vi "Vector Facade.vi"(0 "Data In":T4, 2 "Display State In":T2, 3 "Container State":T3) -> (6 "Data Out":T4, 7 "Display State Out":T2, 8 "Action":T1)   [LabVIEW 2018, in "Vector Function Generator.xctl"]
uses:
  Vector Function Generator.xctl
  Vector Data.ctl
  <vilib>/_xctls/Container State.ctl
  Vector State.ctl
  <vilib>/_xctls/Action.ctl
  <userlib>/_LAVAcr/User_Interface/XControls/Waveform_XControl/Waveform Control.xctl
  <userlib>/_OpenG.lib/comparison/comparison.llb/I32 Changed__ogtk.vi
  <userlib>/_OpenG.lib/comparison/comparison.llb/Boolean Changed__ogtk.vi
  <vilib>/_xctls/XControlSupport.lvlib
panel:
  in  "Order":u16(ring) items=["R then Theta", "Theta then R", "R and Theta"]
  in  "Tab Control":enum32{"R", "Theta", "Plot"}(tab)
  in  "R":waveform(dbl)(xcontrol)
  in  "Theta":waveform(dbl)(xcontrol)
  out "Polar Plot":picture
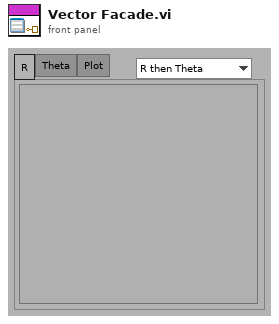
[diagram p1: front panel]
types:
  T1 = typedef "XControlSupport.lvlib/Action.ctl" = cluster{"Data Changed?":bool, "State Changed?":bool, "Action Name":string}
  T2 = typedef "Vector Function Generator.xctl/Vector State.ctl" = cluster{"Current Position":i32, "Show Current Position":bool, "Mode (F=Polar)":bool, "digits":i32, "sf(F) or dp ?":bool, "Units":string}
  T3 = typedef "XControlSupport.lvlib/Container State.ctl" = cluster{"Indicator?":bool, "Run Mode?":bool, " Refnum":refnum<vi>}
  T4 = typedef "Vector Function Generator.xctl/Vector Data.ctl" = waveform(cdb)
  T5 = typedef "Waveform Control.xctl/FP Controls.ctl" = cluster{"Type":T6, "Periods":dbl, "Points":i32, "Offset":dbl, "Amplitdue":dbl, "Phase":dbl, "func":string}
  T6 = typedef "Waveform Control.xctl/Function Types.ctl" = enum16{"Level", "Sine", "Triangle", "Ramp", "Saw Tooth", "Square", "Function"}
  T7 = typedef "LVRectTypeDef.ctl" = cluster{"Left":i16, "Top":i16, "Right":i16, "Bottom":i16}
  T8 = typedef "LVBoundsTypeDef.ctl" = cluster{"Width":u32, "Height":u32}
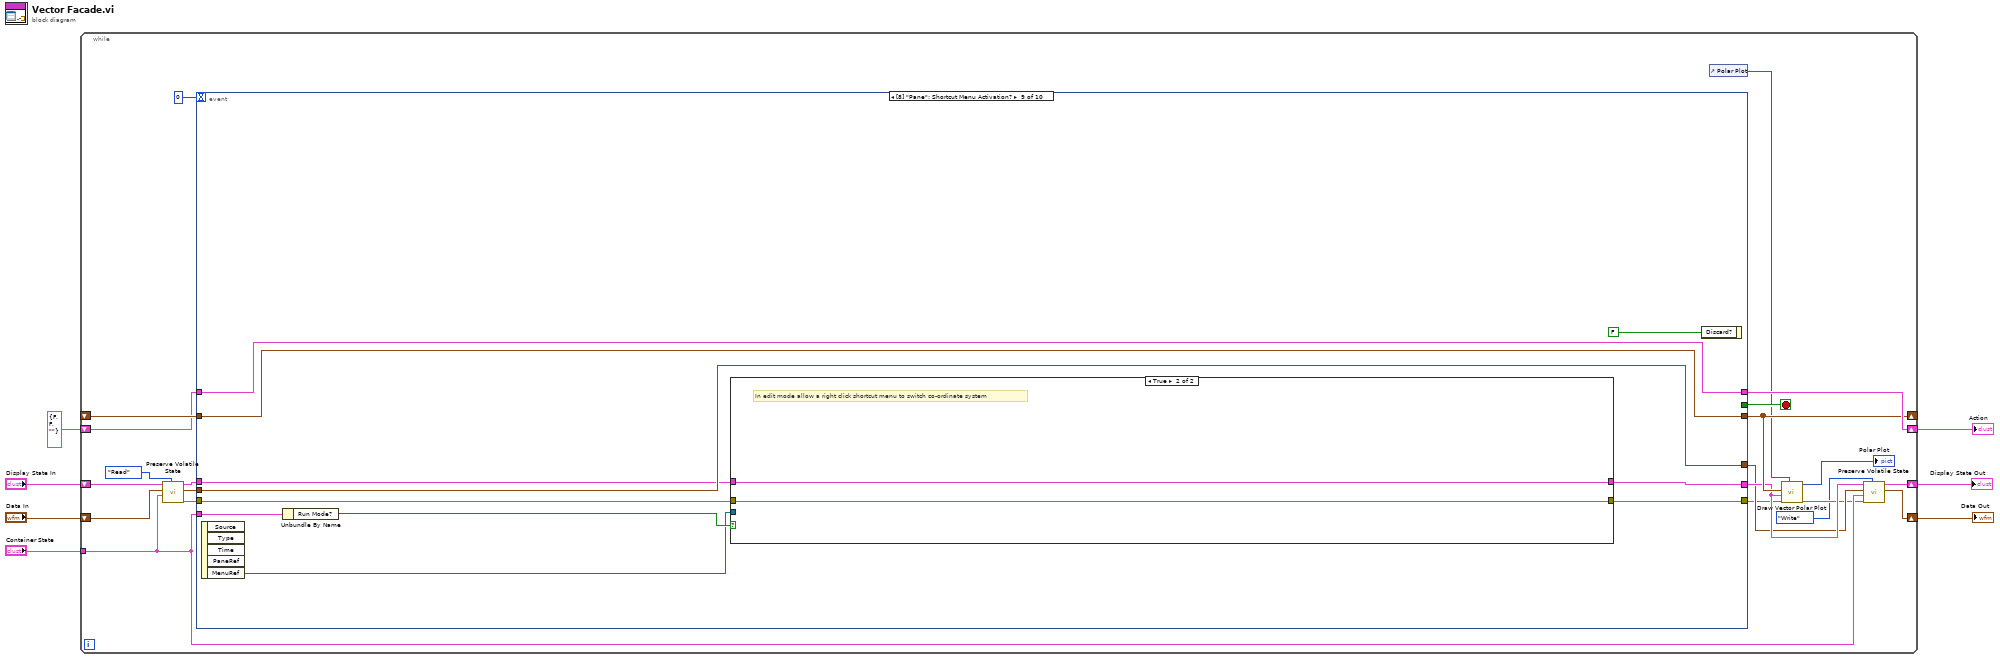
[diagram p0: block diagram]
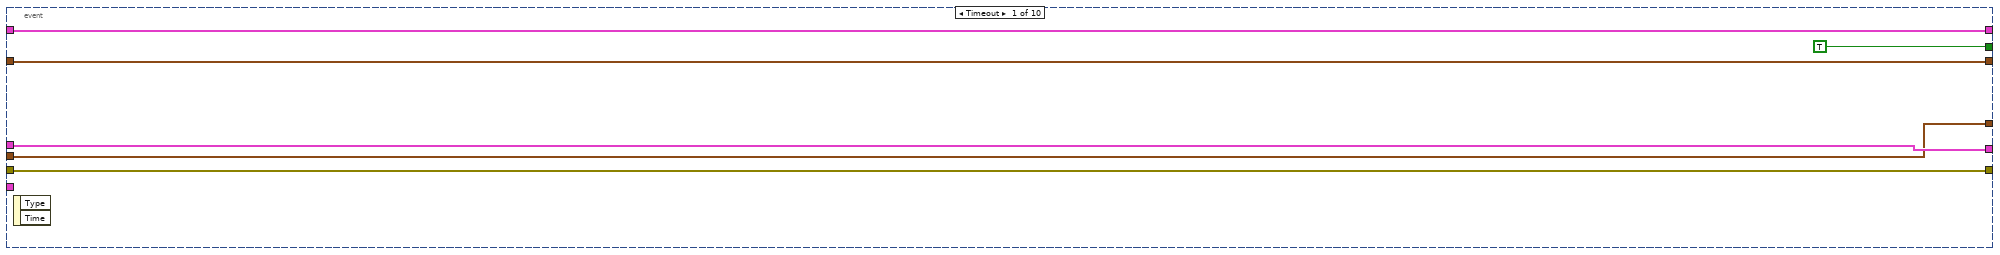
[diagram p2: hidden frame]
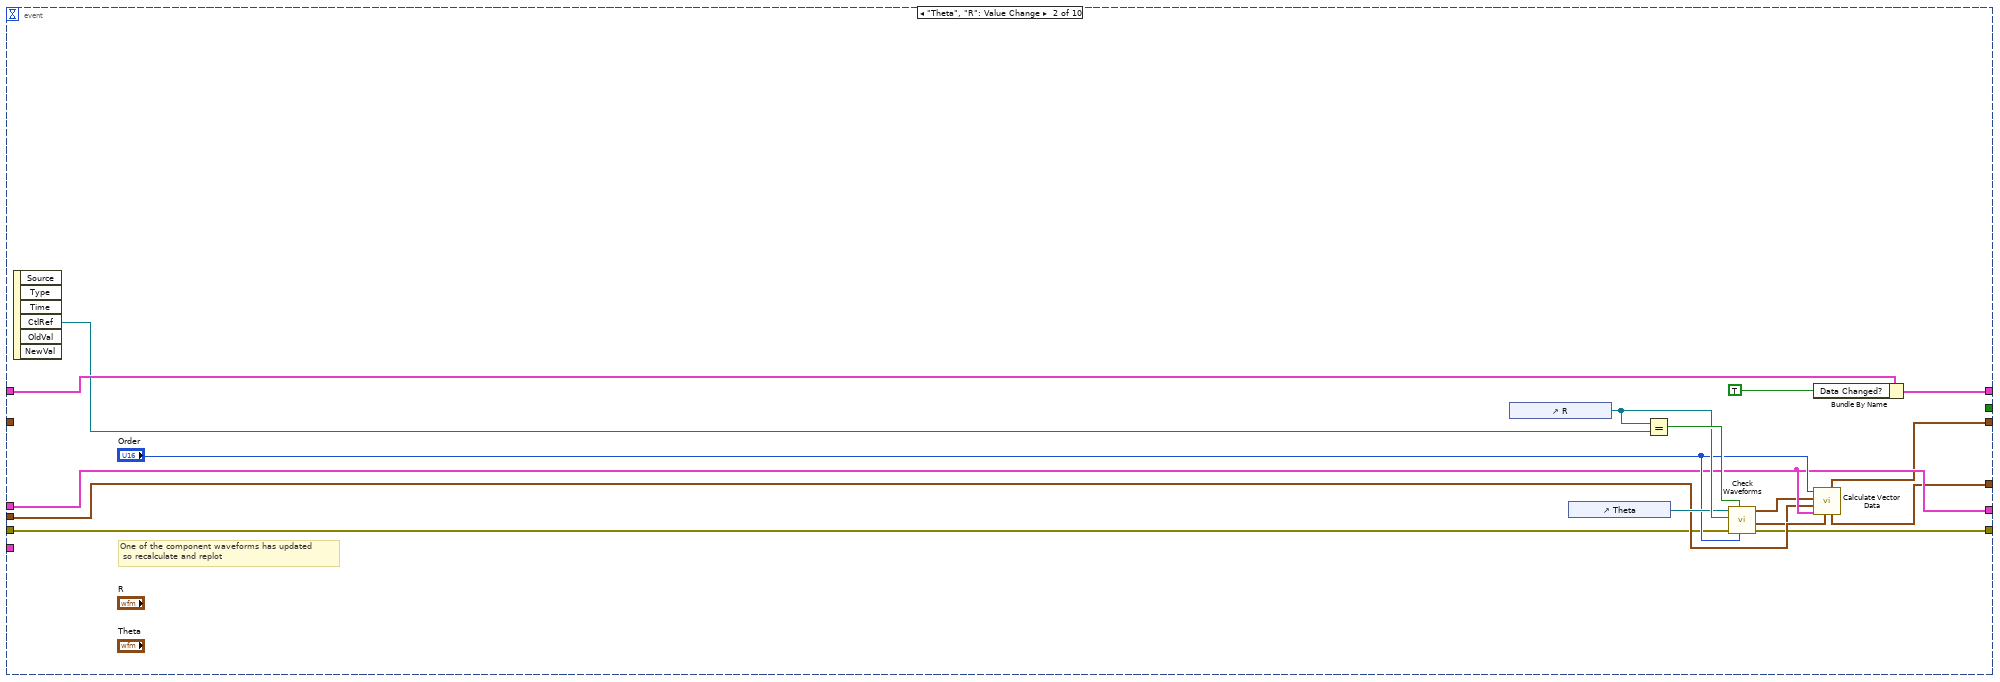
[diagram p3: hidden frame]
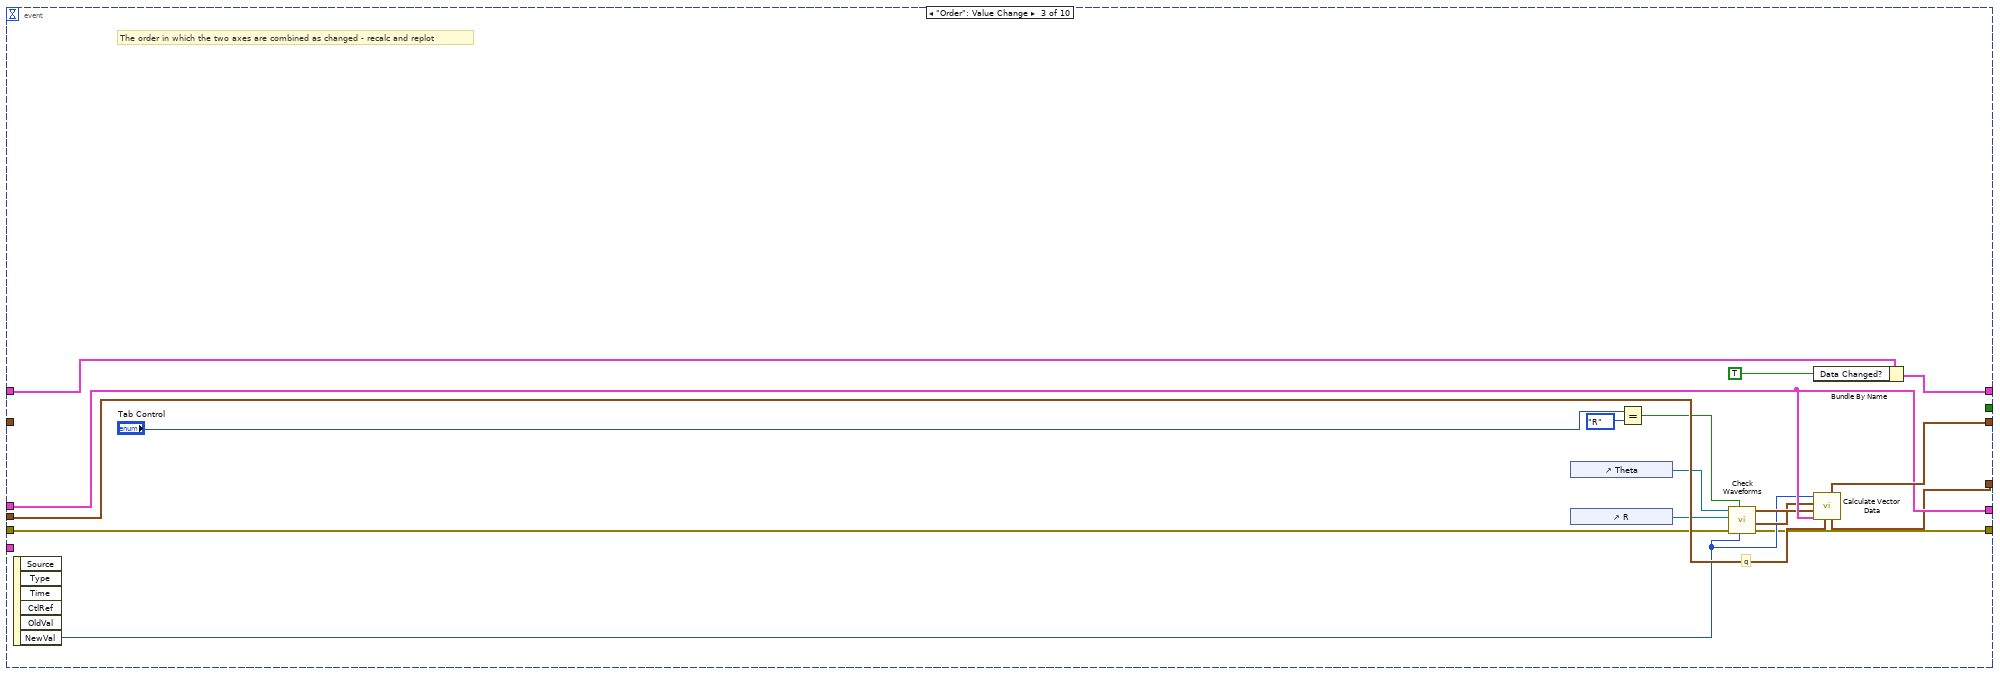
[diagram p4: hidden frame]
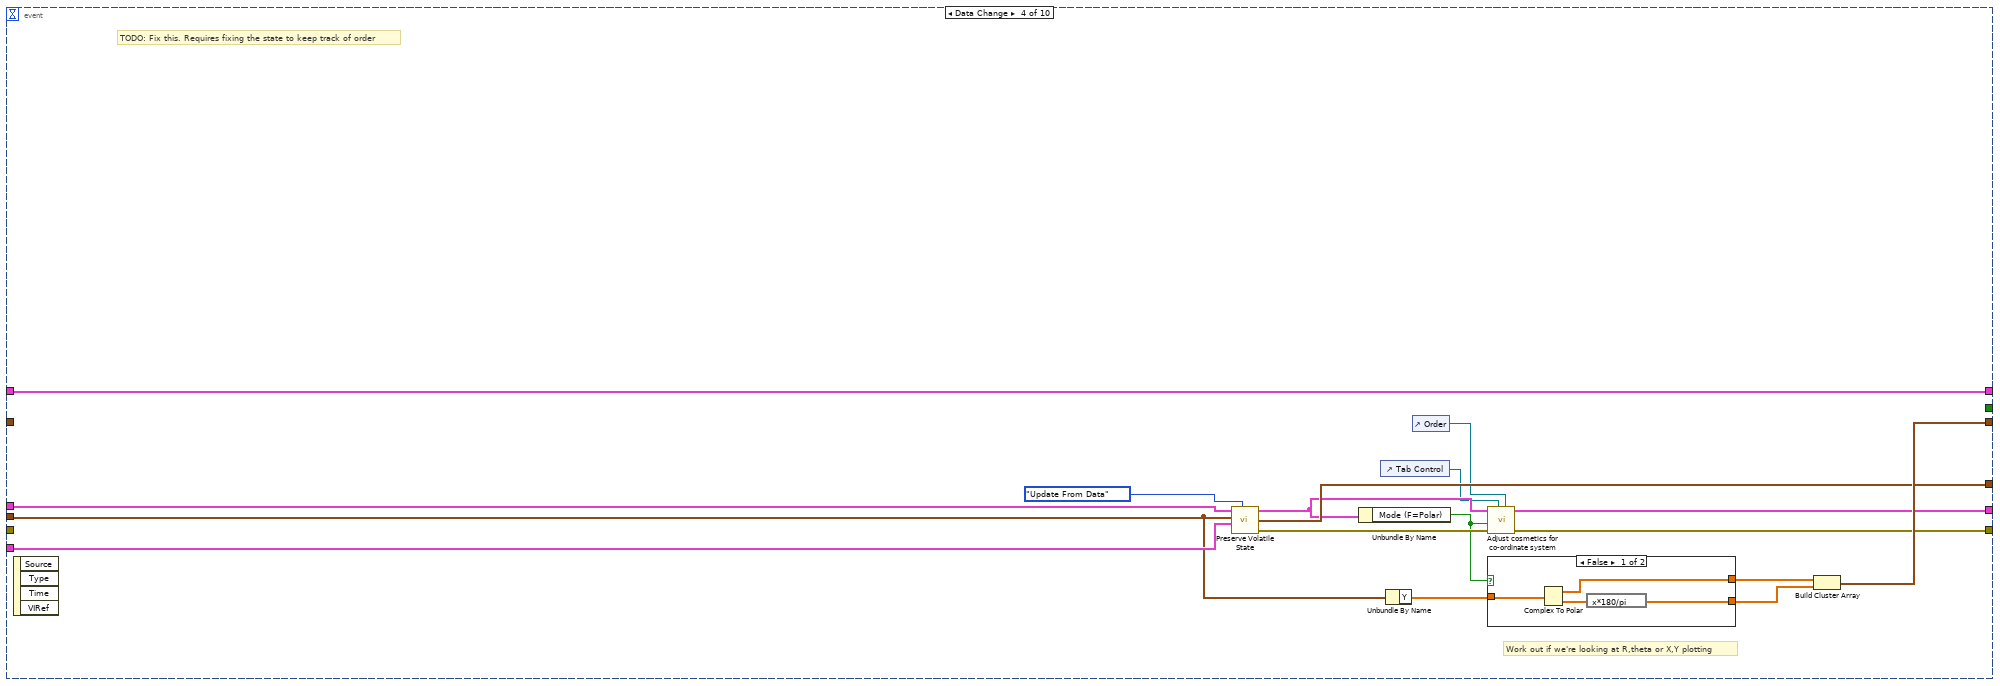
[diagram p5: hidden frame]
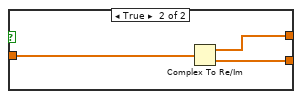
[diagram p6: hidden frame]
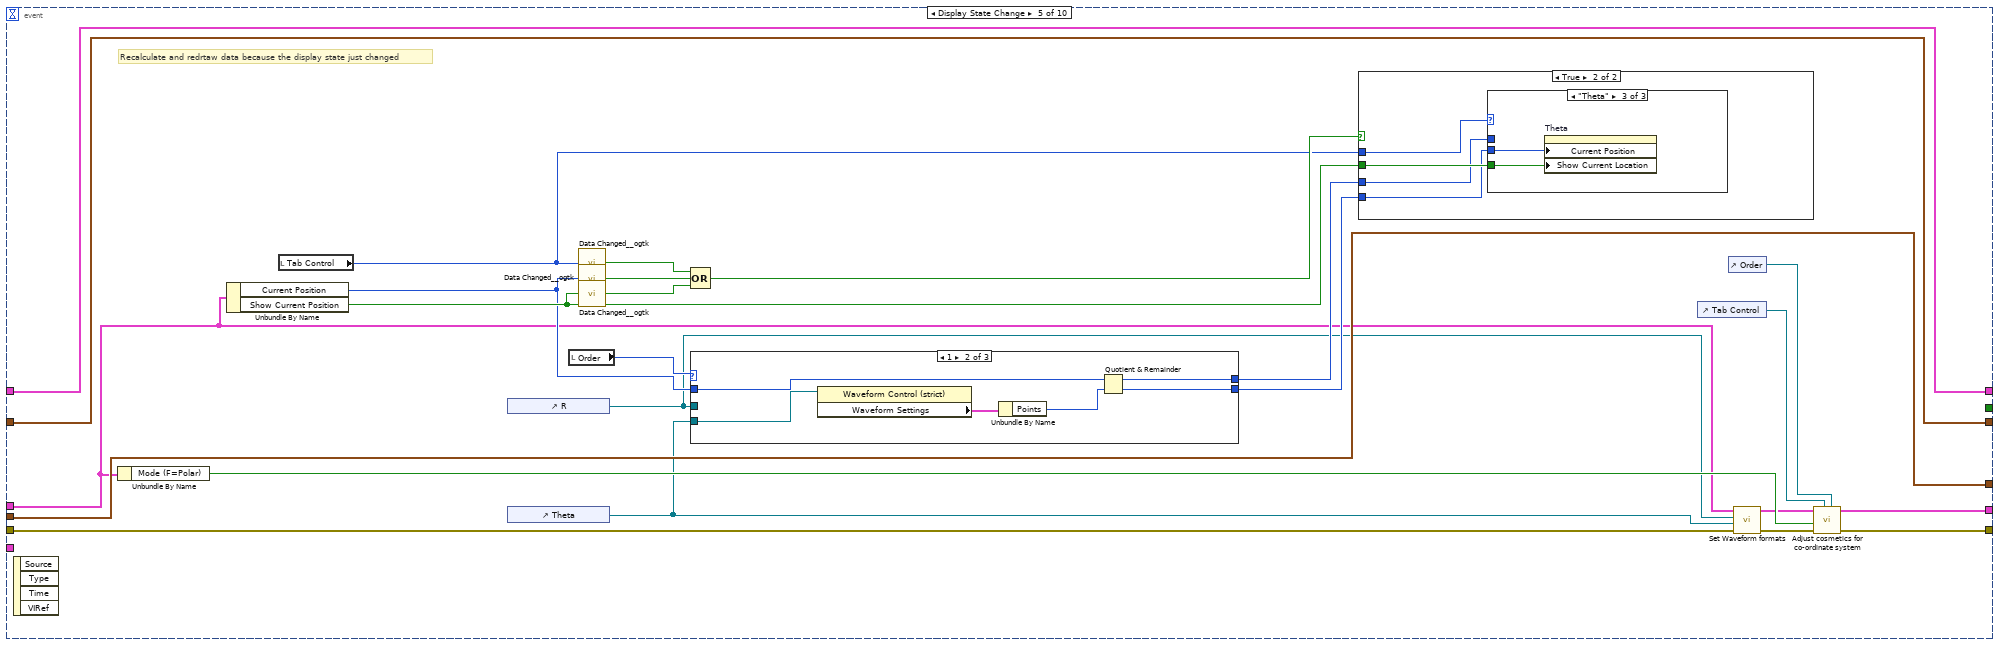
[diagram p7: hidden frame]
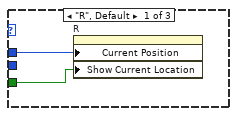
[diagram p9: hidden frame]
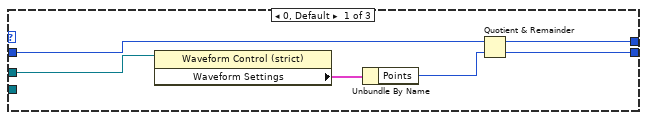
[diagram p11: hidden frame]
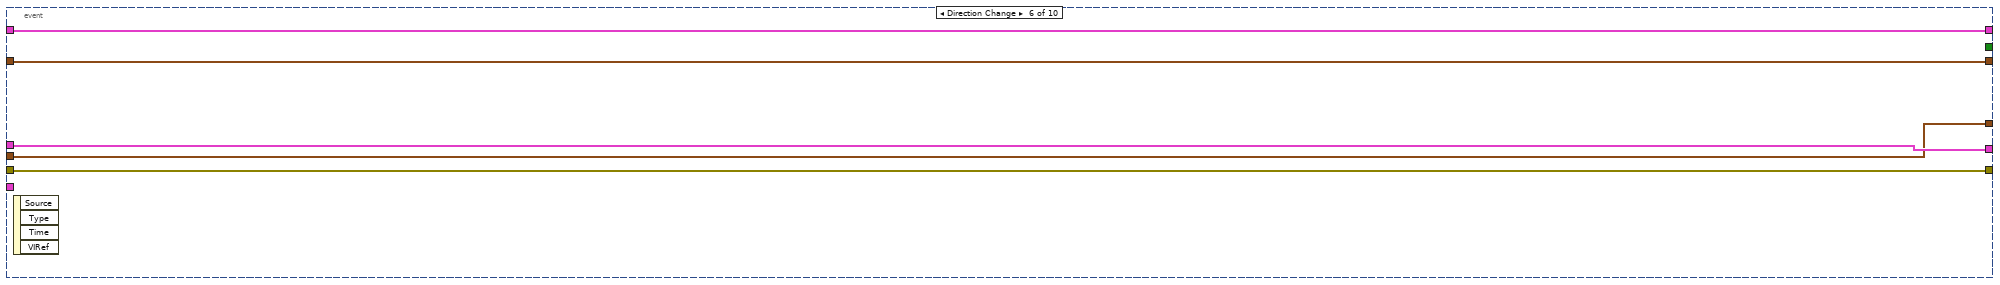
[diagram p13: hidden frame]
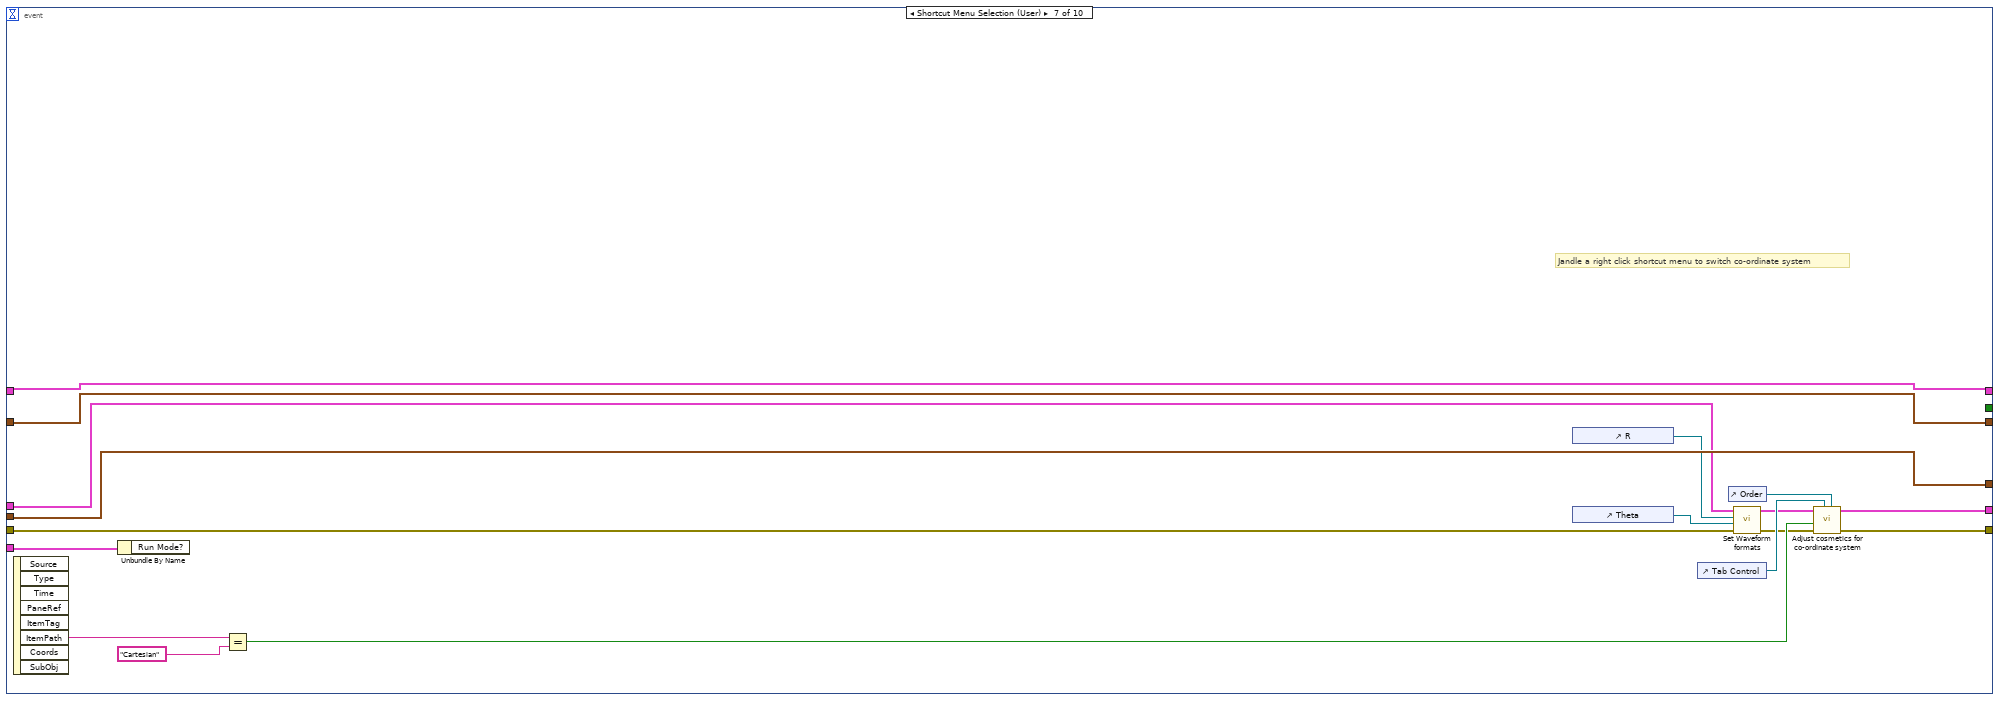
[diagram p14: hidden frame]
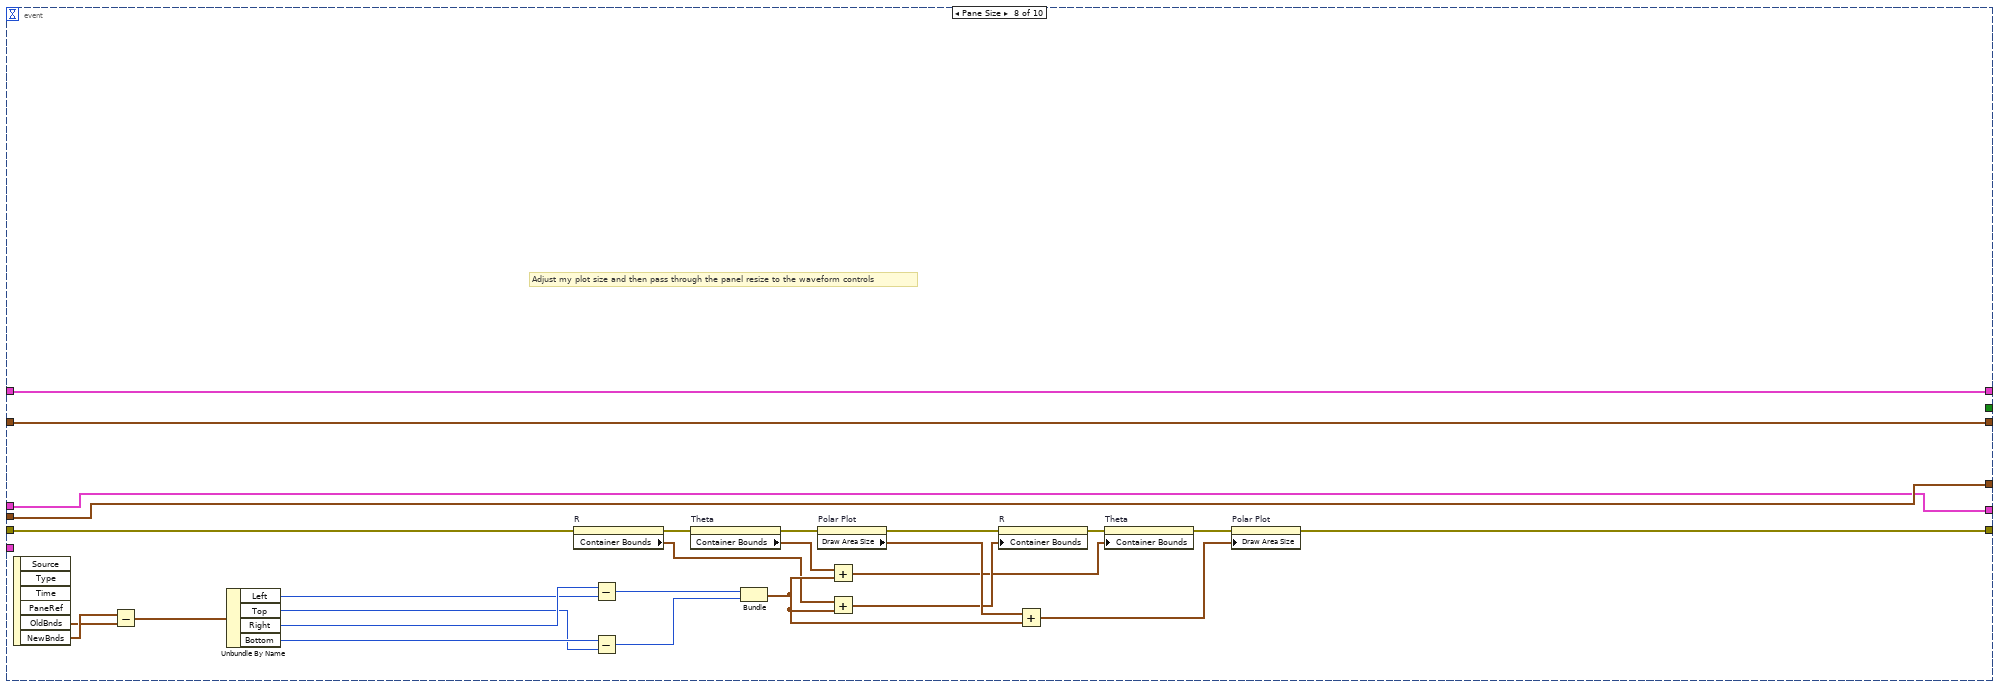
[diagram p15: hidden frame]
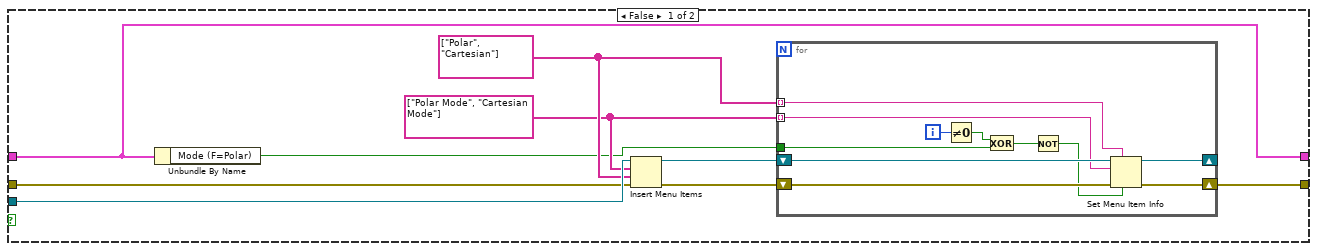
[diagram p16: hidden frame]
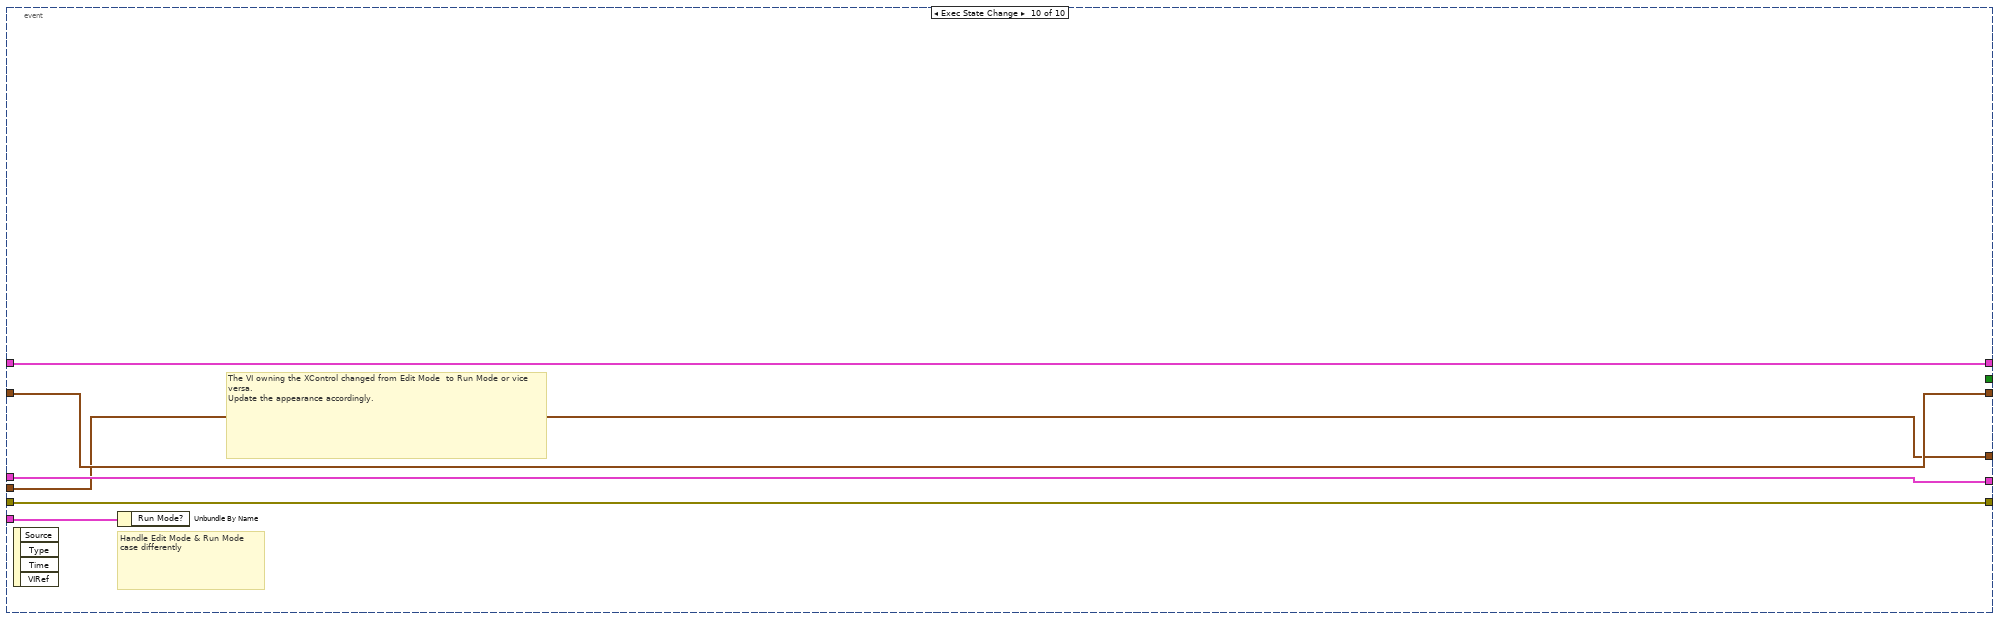
[diagram p17: hidden frame]
diagram:
  n1 = while {
    shift-right: [w14] -> w6
    shift-left: "Display State In" -> [w22]
    tunnel: "Container State" -> [w15]
    shift-right: [w24] -> _
    shift-left: _ -> [w27]
    shift-right: [w25] -> w4
    shift-left: T1 {"Data Changed?"=FALSE, "State Changed?"=FALSE, "Action Name"=""} ("Action") -> [w26]
    shift-right: [w13] -> w1
    shift-left: "Data In" -> [w20]
    stop <- w29 stop-if-true
    n2 = call "Preserve Volatile State.vi"("Operation In"=enum16{"Read", "Write", "Update From Data"}."Read" ("Operation"), "Container State In"=w15, "Waveform In"=w20, "Waveform State In"=w22) -> ("Error Out"=w9:errorcluster, "Waveform Out"=w19:T4, "Waveform State Out"=w21:T2)  [unwired: 1 in, 4 out]
    n3 = event shown="[8] \"Pane\": Shortcut Menu Activation?" {
      selector: _ -> [_ _ _ _ _ _ _ _ _ _]
      dyn-events: _ -> [_ _ _ _ _ _ _ _ _ _]
      timeout: 0 -> [_ _ _ _ _ _ _ _ _ _]
      tunnel: w21 -> [w33 w42 w63 w82 w98 w142 w147 w183 w192 w224]
      tunnel: [w33 w42 w63 w78 w103 w142 w154 w183 w189 w224] -> w17
      tunnel: [TRUE _ _ _ _ _ _ _ _ _] -> w29
      tunnel: w15 -> [_ _ _ w80 _ _ w155 _ w194 w225]
      tunnel: w27 -> [w32 _ _ _ w116 w141 w159 w185 w197 w223]
      tunnel: [w32 w38 w66 w83 w116 w141 w159 w185 w197 w223] -> w24
      tunnel: [w34 w50 w65 w85 w115 w140 w153 w184 w196 w222] -> w25
      tunnel: w26 -> [w34 w51 w54 w85 w115 w140 w153 w184 w196 w222]
      tunnel: [w31 w39 w61 w81 w114 w139 w158 w186 w195 w221] -> w16
      tunnel: w19 -> [w31 w43 w62 w72 w114 w139 w158 w186 w195 w221]
      tunnel: w9 -> [w30 w36 w52 _ w94 w138 w144 w160 w188 w220]
      tunnel: [w30 w37 w53 w74 w93 w138 w143 w161 w187 w220] -> w8
      event Timeout {
        n4 = event-data() -> ()  [unwired: 3 out]
      }
      event "Theta", "R": Value Change {
        # "One of the component waveforms has updated\n so recalculate and replot"
        n5 = event-data() -> ("CtlRef"=w47:refnum<vi>)  [unwired: 6 out]
        n6 = control-ref of="R"() -> (w46:refnum<vi>)
        n7 = control-ref of="Theta"() -> (w45:refnum<vi>)
        n8 = Equal?(x=w46, y=w47) -> (x = y?=w48:bool)
        n9 = call "Check Waveforms.vi"("Order In"="Order", "Tab is on R?"=w48, "Error In (no Error) In"=w36, "X/R In"=w46, "Y/Theta In"=w45) -> ("Error Out"=w37:errorcluster, "Y/Theta  Out"=w40:waveform(dbl), "X/R  Out"=w41:waveform(dbl))  [unwired: 1 in, 3 out]
        n10 = Bundle By Name(cluster=w51, "Data Changed?"=TRUE) -> (w50:T1)
        n11 = call "Calculate Vector Data.vi"("Data In"=w43, "Display State In"=w42, "X or Magnitude In"=w40, "Y or Phase In"=w41, "Order In"="Order") -> ("Data Out"=w39:T4, "R,Theta or X,Y Points Out"=w38:cluster{dbl, dbl}[])  [unwired: 1 in, 4 out]
      }
      event "Order": Value Change {
        # "The order in which the two axes are combined as changed - recalc and replot"
        # "q"
        n12 = event-data() -> ("NewVal"=w55:u16)  [unwired: 6 out]
        n13 = control-ref of="Theta"() -> (w60:refnum<vi>)
        n14 = control-ref of="R"() -> (w59:refnum<vi>)
        n15 = Equal?(x="Tab Control", y=enum32{"R", "Theta", "Plot"}."R") -> (x = y?=w56:bool)
        n16 = call "Check Waveforms.vi"("Order In"=w55, "Tab is on R?"=w56, "Error In (no Error) In"=w52, "X/R In"=w59, "Y/Theta In"=w60) -> ("Error Out"=w53:errorcluster, "Y/Theta  Out"=w57:waveform(dbl), "X/R  Out"=w58:waveform(dbl))  [unwired: 1 in, 3 out]
        n17 = Bundle By Name(cluster=w54, "Data Changed?"=TRUE) -> (w65:T1)
        n18 = call "Calculate Vector Data.vi"("Data In"=w62, "Display State In"=w63, "X or Magnitude In"=w58, "Y or Phase In"=w57, "Order In"=w55) -> ("Data Out"=w61:T4, "R,Theta or X,Y Points Out"=w66:cluster{dbl, dbl}[])  [unwired: 1 in, 4 out]
      }
      event Data Change {
        # "Work out if we're looking at R,theta or X,Y plotting"
        # "TODO: Fix this. Requires fixing the state to keep track of order"
        n19 = event-data() -> ()  [unwired: 5 out]
        n20 = call "Preserve Volatile State.vi"("Operation In"=enum16{"Read", "Write", "Update From Data"}."Update From Data" ("Operation"), "Container State In"=w80, "Waveform In"=w72, "Waveform State In"=w82) -> ("Error Out"=w79:errorcluster, "Waveform Out"=w81:T4, "Waveform State Out"=w77:T2)  [unwired: 1 in, 4 out]
        n21 = Unbundle By Name(w77) -> ("Mode (F=Polar)"=w70:bool)
        n22 = control-ref of="Tab Control"() -> (w76:refnum<vi>)
        n23 = Unbundle By Name(w72) -> ("Y"=w84:cdb[])
        n24 = control-ref of="Order"() -> (w75:refnum<vi>)
        n25 = call "Adjust cosmetics for co-ordinate system.vi"("Ring Refnum In"=w75, "TabCtl Refnum In"=w76, "Error In (no Error) In"=w79, "Coordinate System In"=w70, "Display State In"=w77) -> ("Error In (no Error) Out"=w74:errorcluster, "Display State Out"=w78:T2)  [unwired: 5 out]
        n26 = case shown="False" w70 {
          tunnel: w84 -> [w89 w92]
          tunnel: [w88 w91] -> w73
          tunnel: [w86 w90] -> w71
          frame False {
            n27 = Complex To Polar(r * e^(i*theta)=w89) -> (r=w88:dbl[], theta=w87:dbl[])
            n28 = expression code="x*180/pi"(w87) -> (w86:dbl[])
          }
          frame True {
            n29 = Complex To Re/Im(x + iy=w92) -> (x=w91:dbl[], y=w90:dbl[])
          }
        }
        n30 = Build Cluster Array(w73, w71) -> (w83:cluster{dbl, dbl}[])
      }
      event Display State Change {
        # "Recalculate and redrtaw data because the display state just changed"
        n31 = event-data() -> ()  [unwired: 5 out]
        n32 = Unbundle By Name(w98) -> ("Mode (F=Polar)"=w100:bool)
        n33 = Unbundle By Name(w98) -> ("Current Position"=w108:i32, "Show Current Position"=w112:bool)
        n34 = local read "Tab Control"() -> (w105:enum32{"R", "Theta", "Plot"})
        n35 = control-ref of="R"() -> (w97:refnum<vi>)
        n36 = control-ref of="Theta"() -> (w96:refnum<vi>)
        n37 = local read "Order"() -> (w113:u16)
        n38 = call-poly <userlib>:"Data Changed__ogtk.vi"("I32"=w105) -> ("Changed"=w104:bool)
        n39 = call-poly <userlib>:"Data Changed__ogtk.vi"("I32"=w108) -> ("Changed"=w110:bool)
        n40 = call-poly <userlib>:"Data Changed__ogtk.vi"("Boolean"=w112) -> ("Changed"=w111:bool)
        n41 = Compound Arithmetic op=OR(w104, w110, w111) -> (w109:bool)
        n42 = case shown="1" w113 {
          tunnel: w108 -> [w128 w133 w137]
          tunnel: w96 -> [_ w136 _]
          tunnel: [w127 w132 w137] -> w107
          tunnel: [w126 w131 w137] -> w106
          tunnel: w97 -> [w125 _ _]
          frame 0, Default {
            n43 = property class="Waveform Control (strict)"(reference=w125) -> ("Waveform Settings"=w130:T5)  [unwired: 1 in, 2 out]
            n44 = Unbundle By Name(w130) -> ("Points"=w129:i32)
            n45 = Quotient & Remainder(x=w128, y=w129) -> (x-y*floor(x/y)=w127:i32, floor(x/y)=w126:i32)
          }
          frame 1 {
            n46 = property class="Waveform Control (strict)"(reference=w136) -> ("Waveform Settings"=w135:T5)  [unwired: 1 in, 2 out]
            n47 = Unbundle By Name(w135) -> ("Points"=w134:i32)
            n48 = Quotient & Remainder(x=w133, y=w134) -> (x-y*floor(x/y)=w132:i32, floor(x/y)=w131:i32)
          }
          frame 2 {
          }
        }
        n49 = case shown="True" w109 {
          tunnel: w105 -> [_ w120]
          tunnel: w112 -> [_ w119]
          tunnel: w107 -> [_ w118]
          tunnel: w106 -> [_ w117]
          frame False {
          }
          frame True {
            n50 = case shown="\"Theta\"" w120 {
              tunnel: w119 -> [w122 _ w124]
              tunnel: w118 -> [w121 _ _]
              tunnel: w117 -> [_ _ w123]
              frame "R", Default {
                n51 = property on="R" class="Waveform Control (strict)"("Current Position"=w121, "Show Current Location"=w122) -> ()  [unwired: 2 in, 2 out]
              }
              frame "Plot" {
              }
              frame "Theta" {
                n52 = property on="Theta" class="Waveform Control (strict)"("Current Position"=w123, "Show Current Location"=w124) -> ()  [unwired: 2 in, 2 out]
              }
            }
          }
        }
        n53 = control-ref of="Tab Control"() -> (w102:refnum<vi>)
        n54 = control-ref of="Order"() -> (w101:refnum<vi>)
        n55 = call "Set Waveform formats.vi"("error in (no error)"=w94, "Theta"=w96, "R"=w97, "State In"=w98) -> ("error out"=w95:errorcluster, "State Out"=w99:T2)  [unwired: 6 out]
        n56 = call "Adjust cosmetics for co-ordinate system.vi"("Ring Refnum In"=w101, "TabCtl Refnum In"=w102, "Error In (no Error) In"=w95, "Coordinate System In"=w100, "Display State In"=w99) -> ("Error In (no Error) Out"=w93:errorcluster, "Display State Out"=w103:T2)  [unwired: 3 in, 2 out]
      }
      event Direction Change {
        n57 = event-data() -> ()  [unwired: 5 out]
      }
      event Shortcut Menu Selection (User) {
        # "Jandle a right click shortcut menu to switch co-ordinate system"
        n58 = event-data() -> ("ItemPath"=w157:string)  [unwired: 8 out]
        n59 = Unbundle By Name(w155) -> ()  [unwired: 1 out]
        n60 = Equal?(x=w157, y="Cartesian") -> (x = y?=w150:bool)
        n61 = control-ref of="R"() -> (w145:refnum<vi>)
        n62 = control-ref of="Theta"() -> (w146:refnum<vi>)
        n63 = control-ref of="Tab Control"() -> (w151:refnum<vi>)
        n64 = control-ref of="Order"() -> (w152:refnum<vi>)
        n65 = call "Set Waveform formats.vi"("error in (no error)"=w144, "Theta"=w146, "R"=w145, "State In"=w147) -> ("error out"=w148:errorcluster, "State Out"=w149:T2)  [unwired: 6 out]
        n66 = call "Adjust cosmetics for co-ordinate system.vi"("Ring Refnum In"=w152, "TabCtl Refnum In"=w151, "Error In (no Error) In"=w148, "Coordinate System In"=w150, "Display State In"=w149) -> ("Error In (no Error) Out"=w143:errorcluster, "Display State Out"=w154:T2)  [unwired: 3 in, 2 out]
      }
      event Pane Size {
        # "Adjust my plot size and then pass through the panel resize to the waveform controls"
        n67 = event-data() -> ("OldBnds"=w176:T7, "NewBnds"=w177:T7)  [unwired: 5 out]
        n68 = Subtract(x=w177, y=w176) -> (x-y=w175:T7)
        n69 = Unbundle By Name(w175) -> ("Left"=w173:i16, "Top"=w171:i16, "Right"=w174:i16, "Bottom"=w172:i16)
        n70 = property on="R" class="Waveform Control (strict)"(error in=w160) -> (error out=w182:errorcluster, "Container Bounds"=w167:T8)  [unwired: 1 in, 1 out]
        n71 = Subtract(x=w174, y=w173) -> (x-y=w170:i16)
        n72 = Subtract(x=w172, y=w171) -> (x-y=w169:i16)
        n73 = property on="Theta" class="Waveform Control (strict)"(error in=w182) -> (error out=w181:errorcluster, "Container Bounds"=w166:T8)  [unwired: 1 in, 1 out]
        n74 = Bundle(w170, w169) -> (w168:cluster{i16, i16})  [unwired: 1 out]
        n75 = property on="Polar Plot" class="Pict"(error in=w181) -> (error out=w178:errorcluster, "Draw Area Size"=w165:T8)  [unwired: 1 in, 1 out]
        n76 = Add(x=w166, y=w168) -> (x+y=w163:T8)
        n77 = Add(x=w167, y=w168) -> (x+y=w164:T8)
        n78 = property on="R" class="Waveform Control (strict)"(error in=w178, "Container Bounds"=w164) -> (error out=w179:errorcluster)  [unwired: 1 in, 1 out]
        n79 = Add(x=w165, y=w168) -> (x+y=w162:T8)
        n80 = property on="Theta" class="Waveform Control (strict)"(error in=w179, "Container Bounds"=w163) -> (error out=w180:errorcluster)  [unwired: 1 in, 1 out]
        n81 = property on="Polar Plot" class="Pict"(error in=w180, "Draw Area Size"=w162) -> (error out=w161:errorcluster)  [unwired: 1 in, 1 out]
      }
      event Shortcut Menu Activation? {
        n82 = event-data() -> ("MenuRef"=w191:refnum<k9>)  [unwired: 5 out]
        n83 = Unbundle By Name(w194) -> ("Run Mode?"=w193:bool)
        n84 = case shown="True" w193 {
          tunnel: [w201 w219] -> w189
          tunnel: w192 -> [w201 w219]
          tunnel: w191 -> [w206 _]
          tunnel: w188 -> [w199 w218]
          tunnel: [w198 w218] -> w187
          frame False {
            w203 = string[] ["Polar", "Cartesian"] ("item tags")
            w202 = string[] ["Polar Mode", "Cartesian Mode"] ("item names")
            n85 = Unbundle By Name(w201) -> ("Mode (F=Polar)"=w200:bool)
            n86 = Insert Menu Items(6:w199, 7:w203, 8:w202, 9:w206) -> (0:w205:errorcluster, 3:w204:refnum<k9>)  [unwired: 3 out]
            n87 = for {
              shift-right: [w214] -> _
              shift-left: w204 -> [w217]
              shift-right: [w215] -> w198
              shift-left: w205 -> [w216]
              tunnel: w203 -> [w213] mode=indexing
              tunnel: w202 -> [w210] mode=indexing
              tunnel: w200 -> [w207]
              i -> [w212]
              n88 = Not Equal To 0?(x=w212) -> (x != 0?=w211:bool)
              n89 = Exclusive Or(1:w207, 2:w211) -> (0:w209:bool)
              n90 = Not(x=w209) -> (.not. x?=w208:bool)
              n91 = Set Menu Item Info(6:w208, 7:w213, 8:w216, 10:w210, 11:w217) -> (0:w215:errorcluster, 3:w214:refnum<k9>)  [unwired: 2 out]
            }
          }
          frame True {
            # "In edit mode allow a right click shortcut menu to switch co-ordinate system"
          }
        }
        n92 = event-data("Discard?"=FALSE) -> ()  [unwired: 1 in, 1 out]
      }
      event Exec State Change {
        # "The VI owning the XControl changed from Edit Mode  to Run Mode or vice versa.\nUpdate the appearance accordingly."
        # "Handle Edit Mode & Run Mode\ncase differently"
        n93 = event-data() -> ()  [unwired: 5 out]
        n94 = Unbundle By Name(w225) -> ()  [unwired: 1 out]
      }
    }
    n95 = control-ref of="Polar Plot"() -> (w10:refnum<vi>)
    n96 = call "Draw Vector Polar Plot.vi"("Pcture Refnum In"=w10, "Error In (no Error) In"=w8, "Display State In"=w17, "In"=w24) -> ("Error Out"=w12:errorcluster, "Plot Out"=→"Polar Plot":picture)  [unwired: 1 in, 5 out]
    n97 = call "Preserve Volatile State.vi"("Operation In"=enum16{"Read", "Write", "Update From Data"}."Write" ("Operation"), "Error In (no Error) In"=w12, "Container State In"=w15, "Waveform In"=w16, "Waveform State In"=w17) -> ("Waveform Out"=w13:T4, "Waveform State Out"=w14:T2)  [unwired: 5 out]
  }
  "Display State Out" <- w6
  "Data Out" <- w1
  "Action" <- w4
